vi "DRC91SetSetpoint.vi"(0 "VISA Rsrc":refnum<visa-resource-name>="GPIB0::12::INSTR", 7 "SetPoint":dbl, 11 "error in (no error)":errorcluster) -> (15 "error out":errorcluster)   [LabVIEW 2010]
doc: "Ce VI écrit les paramètres limites de contrôle dans le contrôleur."
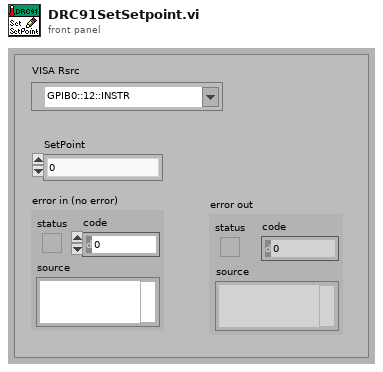
[diagram p1: front panel]
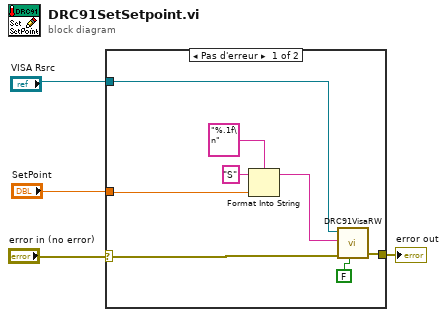
[diagram p0: block diagram]
diagram:
  n1 = case shown="Pas d'erreur" "error in (no error)" {
    selector: "error in (no error)" -> [w10 w13]
    tunnel: "VISA Rsrc" -> [w12 _]
    tunnel: [w11 w13] -> w3
    tunnel: "SetPoint" -> [w5 _]
    frame No Error {
      n2 = Format Into String(format string="%.1f\n" ("chaîne de format"), initial string="S" ("chaîne initiale"), w5) -> (resulting string=w8:string)  [unwired: 1 in, 1 out]
      n3 = call <userlib>:"DRC91VisaRW.vi"("Lecture?(T)"=FALSE, "error in (no error)"=w10, "ChaineCom"=w8, "VISA Rsrc"=w12) -> ("error out"=w11:errorcluster)  [unwired: 3 in, 3 out]
    }
    frame Error {
    }
  }
  "error out" <- w3
